vi "GraphSetting Get PlotName (XY).vi"(8 "error in (no error)":errorcluster caption="エラー入力（エラーなし）", 11 "XYグラフref(in)":refnum<vi>) -> (0 "error out":errorcluster caption="エラー出力", 2 "プロット名称[]":string[](array[string]))   [LabVIEW 2016]
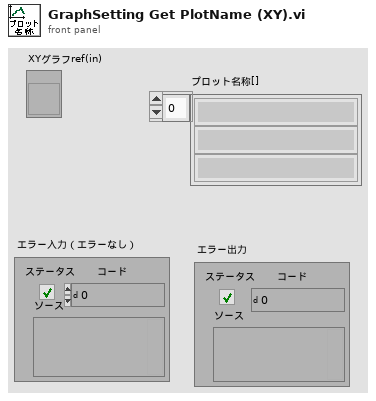
[diagram p1: front panel]
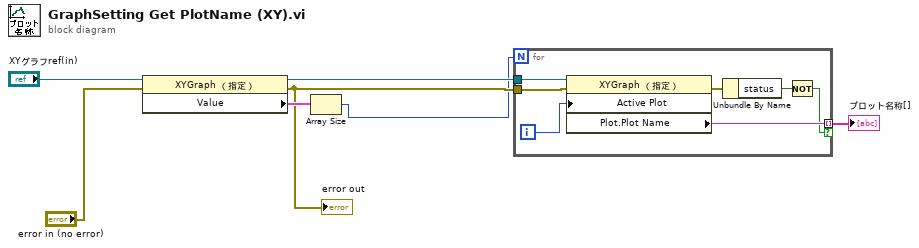
[diagram p0: block diagram]
diagram:
  n1 = property class="XYGraph （指定）"(reference="XYグラフref(in)", error in="error in (no error)") -> (reference out=w5:refnum<vi>, error out=w3:errorcluster, "Value"=w6:cluster{"X":dbl[], "Y":dbl[]}[])
  "error out" <- w3
  n2 = Array Size(array=w6) -> (size(s)=w2:i32)
  n3 = for {
    N: w2 -> [_]
    tunnel: w5 -> [w14]
    tunnel: [w13] -> w7 mode=indexing if=w10
    tunnel: w3 -> [w9]
    i -> [w8]
    n4 = property class="XYGraph （指定）"(reference=w14, error in=w9, "Active Plot"=w8) -> (error out=w12:errorcluster, "Plot.Plot Name"=w13:string)  [unwired: 1 out]
    n5 = Unbundle By Name(w12) -> ("status"=w11:bool)
    n6 = Not(x=w11) -> (.not. x?=w10:bool)
  }
  "プロット名称[]" <- w7
